vi "StartStopPause.vi"() -> ()   [LabVIEW 2020]
panel:
  out "StartStopPauseArray2":bool[][](array[boolean])
  out "StartStopPauseArray1":bool[][](array[boolean])
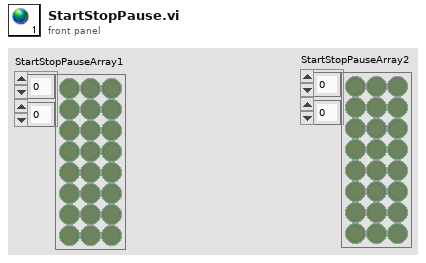
[diagram p1: front panel]
diagram:
